vi "Write data.vi"(8 "error in":errorcluster, 9 "starting address":u16, 10 "register to write":u16, 11 "Modbus master in":refnum<class "Modbus Master.lvclass">) -> (0 "error out":errorcluster, 3 "Modbus master out":refnum<class "Modbus Master.lvclass">)   [LabVIEW 2023, in "RS485.lvlib"]
uses:
  RS485.lvlib
  <vilib>/NI/Modbus Library/API/Master/Modbus Master.lvclass
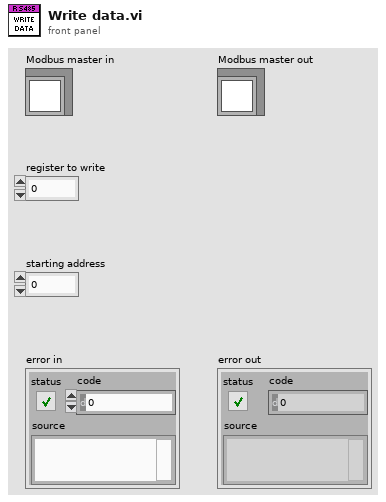
[diagram p1: front panel]
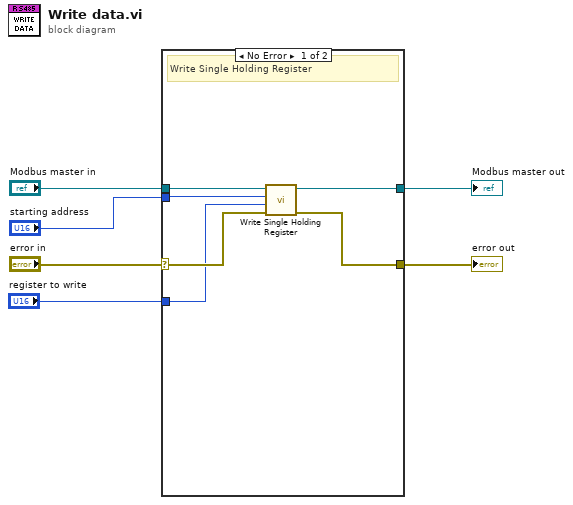
[diagram p0: block diagram]
diagram:
  n1 = case shown="No Error" "error in" {
    selector: "error in" -> [w10 w13]
    tunnel: "Modbus master in" -> [w12 w14]
    tunnel: [w11 w14] -> w3
    tunnel: [w9 w13] -> w2
    tunnel: "starting address" -> [w8 _]
    tunnel: "register to write" -> [w7 _]
    frame No Error {
      # "Write Single Holding Register"
      n2 = call-dynamic "Write Single Holding Register.vi"("error in"=w10, "register to write"=w7, "address"=w8, "Modbus master in"=w12) -> ("error out"=w9:errorcluster, "Modbus master out"=w11:refnum<class "Modbus Master.lvclass">)  [unwired: 6 in]
    }
    frame Error {
      # "Error in Initialization"
    }
  }
  "Modbus master out" <- w3
  "error out" <- w2
